vi "parseEMCY.vi"(8 "error in (no error)":errorcluster, 10 "emergency message":T1, 11 "MotorController in":refnum<class "MotorController.lvclass">) -> (0 "error out":errorcluster, 3 "MotorController out":refnum<class "MotorController.lvclass">)   [LabVIEW 2017, in "MotorController.lvclass"]
uses:
  MotorController.lvclass
  MotorController.lvclass/MotorController.ctl
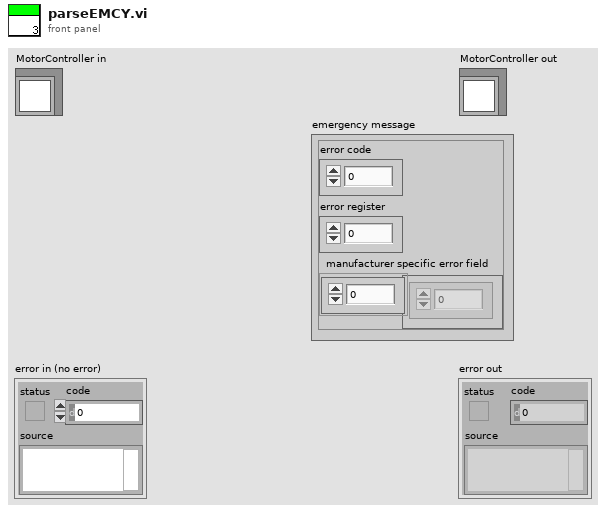
[diagram p1: front panel]
types:
  T1 = cluster{"error code":dbl, "error register":dbl, "manufacturer specific error field":dbl[]}
  T2 = typedef "MotorData.ctl" = cluster{"Velo (RPM)":i32, "MotorTemp(C)":u8, "CtrlTemp(C)":u8, "DcLinkVolt(V)":dbl, "ErrorCode":dbl, "isAlive":bool, "motorControllerState":u16, "motorStatus":T3}
  T3 = typedef "MotorStatus.ctl" = cluster{"isReady":bool, "isOn":bool, "isOperEn":bool, "isFault":bool, "isVoltEn":bool, "targetReached":bool, "isWarning":bool}
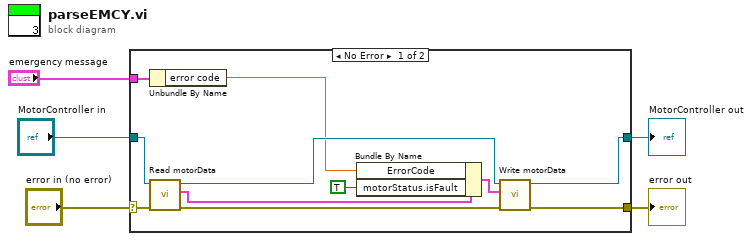
[diagram p0: block diagram]
diagram:
  n1 = case shown="No Error" "error in (no error)" {
    selector: "error in (no error)" -> [w16 w18]
    tunnel: [w10 w18] -> w4
    tunnel: [w9 w17] -> w2
    tunnel: "MotorController in" -> [w15 w17]
    tunnel: "emergency message" -> [w8 _]
    frame No Error {
      n2 = Unbundle By Name(w8) -> ("error code"=w7:dbl)
      n3 = call "Read motorData.vi"("error in (no error)"=w16, "MotorController in"=w15) -> ("error out"=w11:errorcluster, "motorData"=w14:T2, "MotorController out"=w12:refnum<class "MotorController.lvclass">)  [unwired: 7 in]
      n4 = Bundle By Name(cluster=w14, "ErrorCode"=w7, "motorStatus.isFault"=TRUE) -> (w13:T2)
      n5 = call "Write motorData.vi"("error in (no error)"=w11, "motorData"=w13, "MotorController in"=w12) -> ("error out"=w10:errorcluster, "MotorController out"=w9:refnum<class "MotorController.lvclass">)  [unwired: 7 in]
    }
    frame Error {
    }
  }
  "error out" <- w4
  "MotorController out" <- w2
